vi "Drag and Drop.vi"(7 "Mode":T2, 8 "错误输入":errorcluster, 10 "Drag and Drop In":T1, 11 "Listbox Ref":refnum<vi>) -> (0 "错误输出":errorcluster, 2 "Drag and Drop Out":T1, 3 "Dup Listbox Ref":refnum<vi>)   [LabVIEW 2012, in "Listbox Tool.lvlib"]
uses:
  Listbox Tool.lvlib
  Custom Type/Read and Write Mode.ctl
  Custom Type/Drag and Drop.ctl
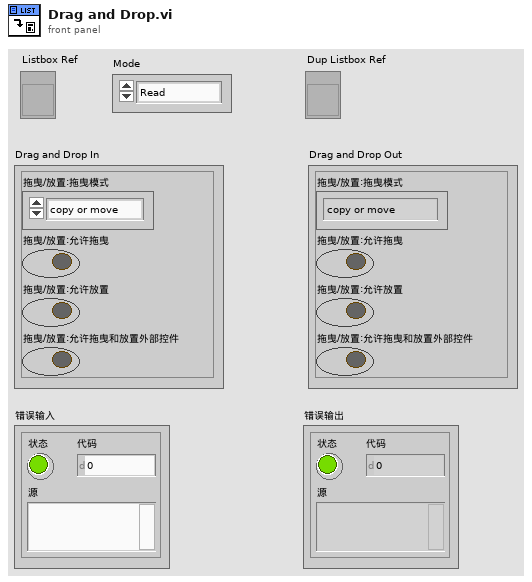
[diagram p1: front panel]
types:
  T1 = typedef "Listbox Tool.lvlib/Drag and Drop.ctl" = cluster{"拖曳/放置:拖曳模式":enum32{"copy or move", "copy only", "move only"}, "拖曳/放置:允许拖曳":bool, "拖曳/放置:允许放置":bool, "拖曳/放置:允许拖曳和放置外部控件":bool}
  T2 = typedef "Listbox Tool.lvlib/Read and Write Mode.ctl" = enum16{"Read", "Write"}
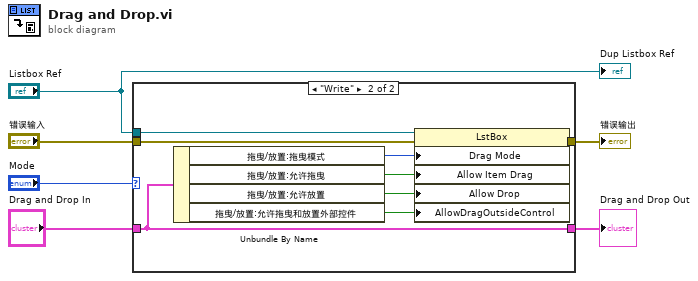
[diagram p0: block diagram]
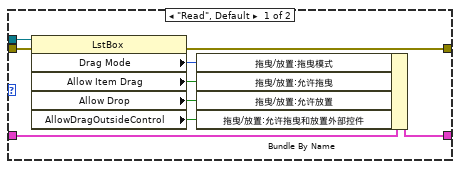
[diagram p2: hidden frame]
diagram:
  n1 = case shown="\"Write\"" "Mode" {
    tunnel: "错误输入" -> [w14 w23]
    tunnel: [w13 w22] -> w5
    tunnel: "Listbox Ref" -> [w15 w21]
    tunnel: "Drag and Drop In" -> [w9 w16]
    tunnel: [w8 w16] -> w1
    frame "Read", Default {
      n2 = property class="LstBox"(reference=w15, error in=w14) -> (error out=w13:errorcluster, "Drag Mode"=w12:enum32{"copy or move", "copy only", "move only"}, "Allow Item Drag"=w11:bool, "Allow Drop"=w10:bool, "AllowDragOutsideControl"=w7:bool)  [unwired: 1 out]
      n3 = Bundle By Name(cluster=w9, "拖曳/放置:拖曳模式"=w12, "拖曳/放置:允许拖曳"=w11, "拖曳/放置:允许放置"=w10, "拖曳/放置:允许拖曳和放置外部控件"=w7) -> (w8:T1)
    }
    frame "Write" {
      n4 = Unbundle By Name(w16) -> ("拖曳/放置:拖曳模式"=w20:enum32{"copy or move", "copy only", "move only"}, "拖曳/放置:允许拖曳"=w19:bool, "拖曳/放置:允许放置"=w18:bool, "拖曳/放置:允许拖曳和放置外部控件"=w17:bool)
      n5 = property class="LstBox"(reference=w21, error in=w23, "Drag Mode"=w20, "Allow Item Drag"=w19, "Allow Drop"=w18, "AllowDragOutsideControl"=w17) -> (error out=w22:errorcluster)  [unwired: 1 out]
    }
  }
  "错误输出" <- w5
  "Drag and Drop Out" <- w1
  "Dup Listbox Ref" <- "Listbox Ref"
